vi "ConstructTestInstructionArray.vi"(8 "Pixel Size":dbl, 9 "Sample Height":dbl, 10 "Sample Width":dbl) -> (3 "Array":T1(array[ring]))   [LabVIEW 2024]
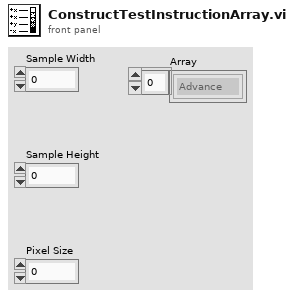
[diagram p1: front panel]
types:
  T1 = enum16{"Advance", "Nothing", "Reverse", "Drop", "Finish"}[]
  T2 = enum16{"Advance", "Nothing", "Reverse", "Drop", "Finish"}
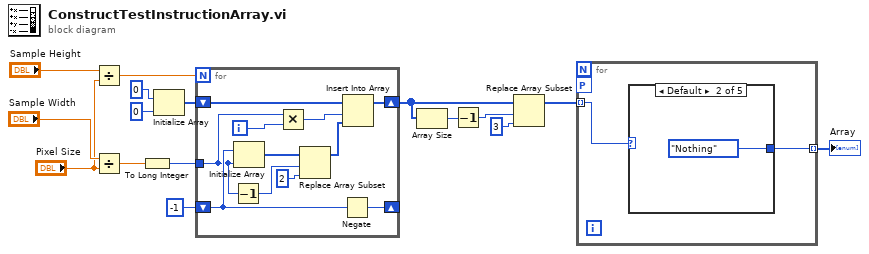
[diagram p0: block diagram]
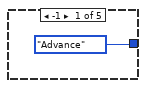
[diagram p2: hidden frame]
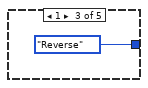
[diagram p3: hidden frame]
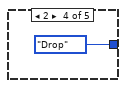
[diagram p4: hidden frame]
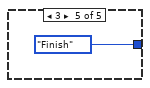
[diagram p5: hidden frame]
diagram:
  n1 = Divide(x="Sample Height", y="Pixel Size") -> (x/y=w5:dbl)
  n2 = Divide(x="Sample Width", y="Pixel Size") -> (x/y=w4:dbl)
  n3 = To Long Integer(number=w4) -> (32bit integer=w3:i32)
  n4 = Initialize Array(0 ("element"), 0 ("dimension size")) -> (w9:i32[])
  n5 = for {
    N: w5 -> [_]
    tunnel: w3 -> [w17]
    shift-right: [w20] -> _
    shift-left: -1 ("Numeric 2") -> [w19]
    shift-right: [w27] -> w13
    shift-left: w9 -> [w26]
    i -> [w18]
    n6 = Decrement(x=w17) -> (x-1=w23:i32)
    n7 = Initialize Array(w19, w17) -> (w24:i32[])
    n8 = Multiply(x=w17, y=w18) -> (x*y=w25:i32)
    n9 = Replace Array Subset(array=w24, new element=2 ("new element/subarray"), index=w23) -> (w21:i32[])
    n10 = Negate(x=w19) -> (-x=w20:i32)
    n11 = Insert Into Array(array=w26, index=w25, new element=w21) -> (w27:i32[])
  }
  n12 = Array Size(array=w13) -> (size(s)=w14:i32)
  n13 = Decrement(x=w14) -> (x-1=w16:i32)
  n14 = Replace Array Subset(array=w13, new element=3 ("new element/subarray"), index=w16) -> (w2:i32[])
  n15 = for {
    tunnel: w2 -> [w29] mode=indexing
    tunnel: [w28] -> w1 mode=indexing
    workers-P: _ -> [_]
    n16 = case shown="Default" w29 {
      tunnel: [T2."Advance" T2."Nothing" T2."Reverse" T2."Drop" T2."Finish"] -> w28
      frame -1 {
      }
      frame Default {
      }
      frame 1 {
      }
      frame 2 {
      }
      frame 3 {
      }
    }
  }
  "Array" <- w1
